vi "Close Communications.vi"(8 "error in (no error)":errorcluster, 10 "Final Stop?":bool, 11 "TCPIP Communications in":refnum<class "TCPIP Communications.lvclass">) -> (0 "error out":errorcluster, 3 "TCPIP Communications out":refnum<class "TCPIP Communications.lvclass">)   [LabVIEW 2015, in "TCPIP Communications Framework.lvlib" / "TCPIP Communications.lvclass"]
uses:
  TCPIP Communications.lvclass
  TCPIP Communications.lvclass/TCPIP Communications.ctl
  <vilib>/ActorFramework/Actor/Actor.lvclass/Actor.ctl
  <vilib>/ActorFramework/Message Enqueuer/Message Enqueuer.lvclass/Message Enqueuer.ctl
  <vilib>/ActorFramework/Message Enqueuer/Init from Existing Queue.vi
  <vilib>/ActorFramework/Message Enqueuer/Enqueue.vi
  <vilib>/ActorFramework/Message Priority Queue/Priority Enqueue.vi
  <vilib>/ActorFramework/Message Enqueuer/Message Enqueuer.lvclass
  TCPIP Communications Messages/Open Transmission Msg/Open Transmission Msg.lvclass
  TCPIP Communications Messages/Open Reception Msg/Open Reception Msg.lvclass
  <vilib>/ActorFramework/Actor/Actor.lvclass
  Utilities/Status Messaging.llb/Status Messaging.lvlib
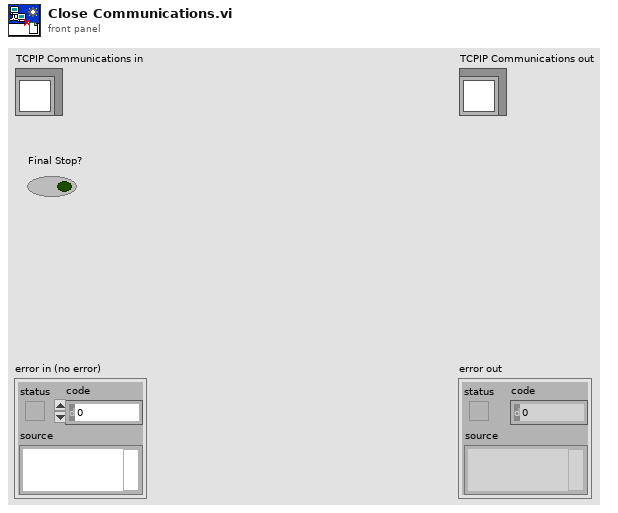
[diagram p1: front panel]
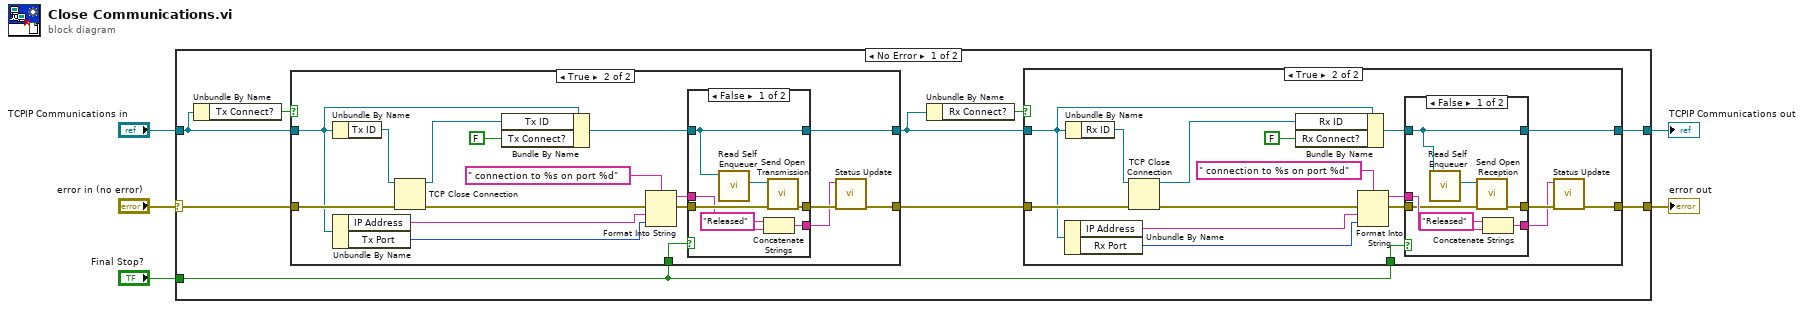
[diagram p0: block diagram]
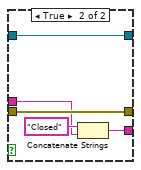
[diagram p3: hidden frame]
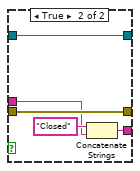
[diagram p5: hidden frame]
diagram:
  n1 = case shown="No Error" "error in (no error)" {
    selector: "error in (no error)" -> [w12 w77]
    tunnel: [w8 w77] -> w4
    tunnel: [w9 w76] -> w2
    tunnel: "TCPIP Communications in" -> [w14 w76]
    tunnel: "Final Stop?" -> [w7 _]
    frame No Error {
      n2 = Unbundle By Name(w14) -> ("Tx Connect?"=w13:bool)
      n3 = case shown="True" w13 {
        tunnel: w14 -> [w46 w55]
        tunnel: [w46 w60] -> w10
        tunnel: w12 -> [w47 w63]
        tunnel: [w47 w62] -> w6
        tunnel: w7 -> [_ w59]
        frame False {
        }
        frame True {
          n4 = Unbundle By Name(w55) -> ("Tx ID"=w57:refnum<k5>)
          n5 = Unbundle By Name(w55) -> ("IP Address"=w54:string, "Tx Port"=w53:u16)
          n6 = TCP Close Connection(connection ID=w57, error in (no error)=w63) -> (connection ID out=w56:refnum<k5>, error out=w52:errorcluster)  [unwired: 1 in]
          n7 = Bundle By Name(cluster=w55, "Tx ID"=w56, "Tx Connect?"=FALSE ("connected?")) -> (w61:refnum<class "TCPIP Communications.lvclass">)
          n8 = Format Into String(format string=" connection to %s on port %d" ("initial string"), error in=w52, w54, w53) -> (resulting string=w50:string, error out=w51:errorcluster)  [unwired: 1 in]
          n9 = case shown="False" w59 {
            tunnel: [w69 w74] -> w62
            tunnel: w51 -> [w68 w74]
            tunnel: w61 -> [w67 w75]
            tunnel: [w67 w75] -> w60
            tunnel: w50 -> [w66 w71]
            tunnel: [w64 w72] -> w49
            frame False {
              n10 = call <vilib>:"Read Self Enqueuer.vi"("Actor"=w67) -> ("Self Enqueuer"=w70:refnum<class "Message Enqueuer.lvclass">)  [unwired: 10 in]
              n11 = Concatenate Strings("Released" ("string"), w66) -> (w64:string)
              n12 = call "Send Open Transmission.vi"("error in (no error)"=w68, "Message Enqueuer"=w70) -> ("error out"=w69:errorcluster)  [unwired: 8 in, 1 out]
            }
            frame True {
              n13 = Concatenate Strings("Closed" ("string"), w71) -> (w72:string)
            }
          }
          n14 = call "Status Update.vi"("Status Update"=w49) -> ()  [unwired: 9 in, 2 out]
        }
      }
      n15 = Unbundle By Name(w10) -> ("Rx Connect?"=w11:bool)
      n16 = case shown="True" w11 {
        tunnel: w10 -> [w15 w26]
        tunnel: [w15 w31] -> w9
        tunnel: w6 -> [w16 w33]
        tunnel: [w16 w25] -> w8
        tunnel: w7 -> [_ w30]
        frame False {
        }
        frame True {
          n17 = Unbundle By Name(w26) -> ("IP Address"=w21:string, "Rx Port"=w20:u16)
          n18 = Unbundle By Name(w26) -> ("Rx ID"=w28:refnum<k5>)
          n19 = TCP Close Connection(connection ID=w28, error in (no error)=w33) -> (connection ID out=w27:refnum<k5>, error out=w23:errorcluster)  [unwired: 1 in]
          n20 = Bundle By Name(cluster=w26, "Rx ID"=w27, "Rx Connect?"=FALSE ("connected?")) -> (w32:refnum<class "TCPIP Communications.lvclass">)
          n21 = Format Into String(format string=" connection to %s on port %d" ("initial string"), error in=w23, w21, w20) -> (resulting string=w19:string, error out=w22:errorcluster)  [unwired: 1 in]
          n22 = case shown="False" w30 {
            tunnel: [w35 w44] -> w24
            tunnel: w32 -> [w40 w45]
            tunnel: [w40 w45] -> w31
            tunnel: w22 -> [w36 w44]
            tunnel: w19 -> [w38 w42]
            tunnel: [w37 w41] -> w18
            frame False {
              n23 = call <vilib>:"Read Self Enqueuer.vi"("Actor"=w40) -> ("Self Enqueuer"=w34:refnum<class "Message Enqueuer.lvclass">)  [unwired: 10 in]
              n24 = call "Send Open Reception.vi"("error in (no error)"=w36, "Message Enqueuer"=w34) -> ("error out"=w35:errorcluster)  [unwired: 8 in, 1 out]
              n25 = Concatenate Strings("Released" ("string"), w38) -> (w37:string)
            }
            frame True {
              n26 = Concatenate Strings("Closed" ("string"), w42) -> (w41:string)
            }
          }
          n27 = call "Status Update.vi"("error in (no error)"=w24, "Status Update"=w18) -> ("error out"=w25:errorcluster)  [unwired: 8 in, 1 out]
        }
      }
    }
    frame Error {
    }
  }
  "error out" <- w4
  "TCPIP Communications out" <- w2
